vi "Receptor PSK.vi"() -> ()   [LabVIEW 2016]
uses:
  <vilib>/addons/Modulation/Digital/Support/Controls/Pack Bits Parameters.ctl
  <vilib>/addons/Modulation/Analog/support/mod_Set Error Source.vi
  <vilib>/addons/Modulation/Analog/support/Validators/mod_Fractional Resample Validate.vi
  <vilib>/addons/Modulation/Analog/support/Validators/mod_Check Flush State.vi
  <vilib>/addons/Modulation/Analog/support/mod_FractionalResampler.vi
  <vilib>/addons/Modulation/Analog/support/mod_Integer Rate Interpolation.vi
  <vilib>/addons/Modulation/Analog/support/Validators/mod_Validate Complex Waveform.vi
  <vilib>/addons/Modulation/Analog/support/mod_PerformResampling.vi
  <vilib>/addons/Modulation/Analog/support/Validators/mod_WFErrorHandler.vi
  <vilib>/addons/Modulation/Digital/Support/Common/Validators/mod_Generate Filter Coefficients Validate.vi
  <vilib>/addons/Modulation/Digital/General/subVIs/mod_Generate Filter Coefficients.vi
  <instrlib>/niUSRP/niUSRP Fetch Rx Data (CDB Cluster).vi
  <vilib>/addons/Modulation/Digital/General/MT Generate PSK System Parameters(M).vi
  <vilib>/addons/Modulation/Digital/General/MT Generate PSK Synchronization Parameters (bit array).vi
  <vilib>/Utility/error.llb/Error Cluster From Error Code.vi
  <vilib>/addons/Modulation/Analog/support/mod_Resampling Factors.vi
  <vilib>/addons/Modulation/Analog/support/mod_ResamplingFilter.vi
  <vilib>/addons/Modulation/Analog/support/mod_Generate Integer Interpolation Filter.vi
  <instrlib>/niUSRP/niUSRP Fetch Rx Data (CDB WDT).vi
  <vilib>/measure/maspectr.llb/FFT Spectrum (Mag-Phase) for 1 Chan (CDB).vi
  <vilib>/addons/Modulation/niDMT.lvlib
  <vilib>/addons/Modulation/niAMT.lvlib
  <vilib>/measure/NI_MAPro.lvlib
panel:
  in  "Header":u32=10 format="%b"
  out "Symbol rate":dbl
  out "output bit stream":i8[](array[numeric])
  out "Magnitude Spectrum":cluster{"f0":dbl, "df":dbl, "magnitude":dbl[]}(graph)={"f0"=-100000.0, "df"=20.0, "magnitude"=[]}
  out "Acquired Signal":waveform(dbl)[](graph)
  out "Frame Size [samples]":i64=20000
  in  "Acq Duration [sec]":dbl=0.01 format="%#.6p"
  in  "autoscale":bool
  out "Constellation Graph":T1(graph)
  in  "stop":bool
  out "measurements":T2={"frequency offset (Hz)"=-11.93165072236316, "frequency drift (Hz)"=0.08770196207837619, "phase offset (deg)"=52.673364140832604} {"phase offset (deg)" format="%.2f"; "frequency drift (Hz)" format="%.2f"; "frequency offset (Hz)" format="%.2f"}
  in  "filter parameters":T3={"Alpha"=0.5, "Filter Length"=6, "TX Filter"=enum."Root Raised Cos"} {"Alpha" format="%.2f"}
  out "Gain [dB] (actual)":dbl=12.0 format="%#.6p"
  out "Carrier Frequency \n[Hz] (actual)":dbl=915000000.0 format="%#.6p"
  out "IQ Sampling\nRate [S/sec] (actual)":dbl=500000.0 format="%#.6p"
  in  "Active Antenna":string(combo)="RX1"
  in  "Gain [dB]":dbl=12.0 format="%#.6p"
  in  "Carrier\nFrequency [Hz]":dbl=915000000.0 format="%#.6p"
  in  "IQ Sampling\nRate [S/sec]":dbl=500000.0 format="%#.6p"
  out "session handle out":refnum<k15>
  in  "error in (no error)":errorcluster
  in  "device names":refnum<k15>
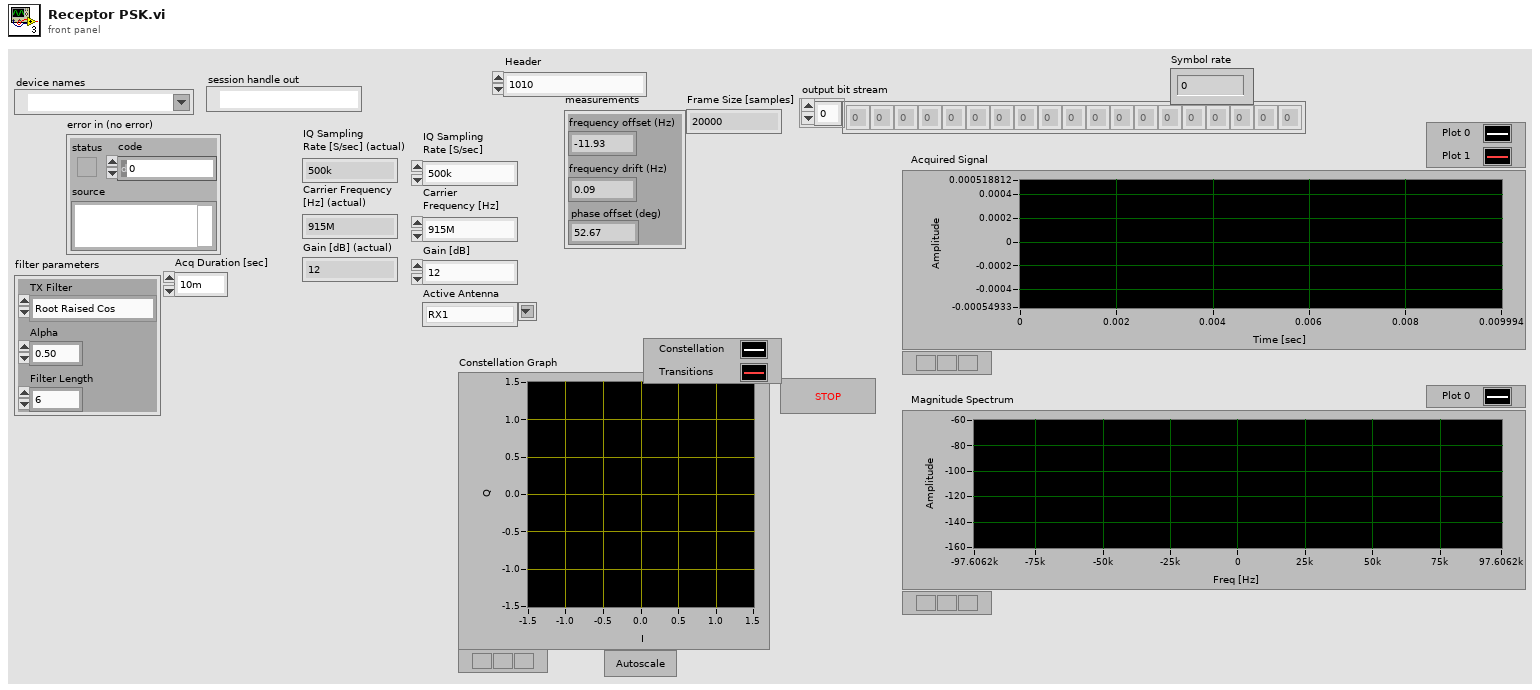
[diagram p1: front panel]
types:
  T1 = cluster{"Decimated Array":dbl[], "Decimated Array":dbl[]}[]
  T2 = cluster{"frequency offset (Hz)":dbl, "frequency drift (Hz)":dbl, "phase offset (deg)":dbl}
  T3 = cluster{"Alpha":dbl, "Filter Length":i32, "TX Filter":enum16{"none", "Raised Cosine", "Root Raised Cos", "Gaussian"}}
  T4 = typedef "niDMT.lvlib/Pack Bits Parameters.ctl" = enum16{"Unsigned", "Signed"}
  T5 = enum16{"FSK", "PSK", "QAM", "MSK", "PAM", "ASK", "CPM"}
  T6 = enum16{"none", "Raised Cosine", "Root Raised Cos", "Gaussian"}
  T7 = cluster{"samples per symbol (16)":i32, "symbol map":cdb[], "differential PSK":enum16{"disable", "enable"}, "PSK type":u16}
  T8 = cluster{"expected sync location (symbols)":i32, "sync sequence":cdb[], "sync location uncertainty (symbols)":i32, "sync indent (symbols)":i32}
  T9 = cluster{"dB On (F)":bool, "unwrap phase (F)":bool, "convert to degree (F)":bool}
  T10 = typedef "niAMT.lvlib/Complex Data Waveform.ctl" = cluster{"t0":dbl, "dt":dbl, "Y":cdb[]}
  T11 = cluster{"constellation":dbl[], "oversampled data":dbl[]}[]
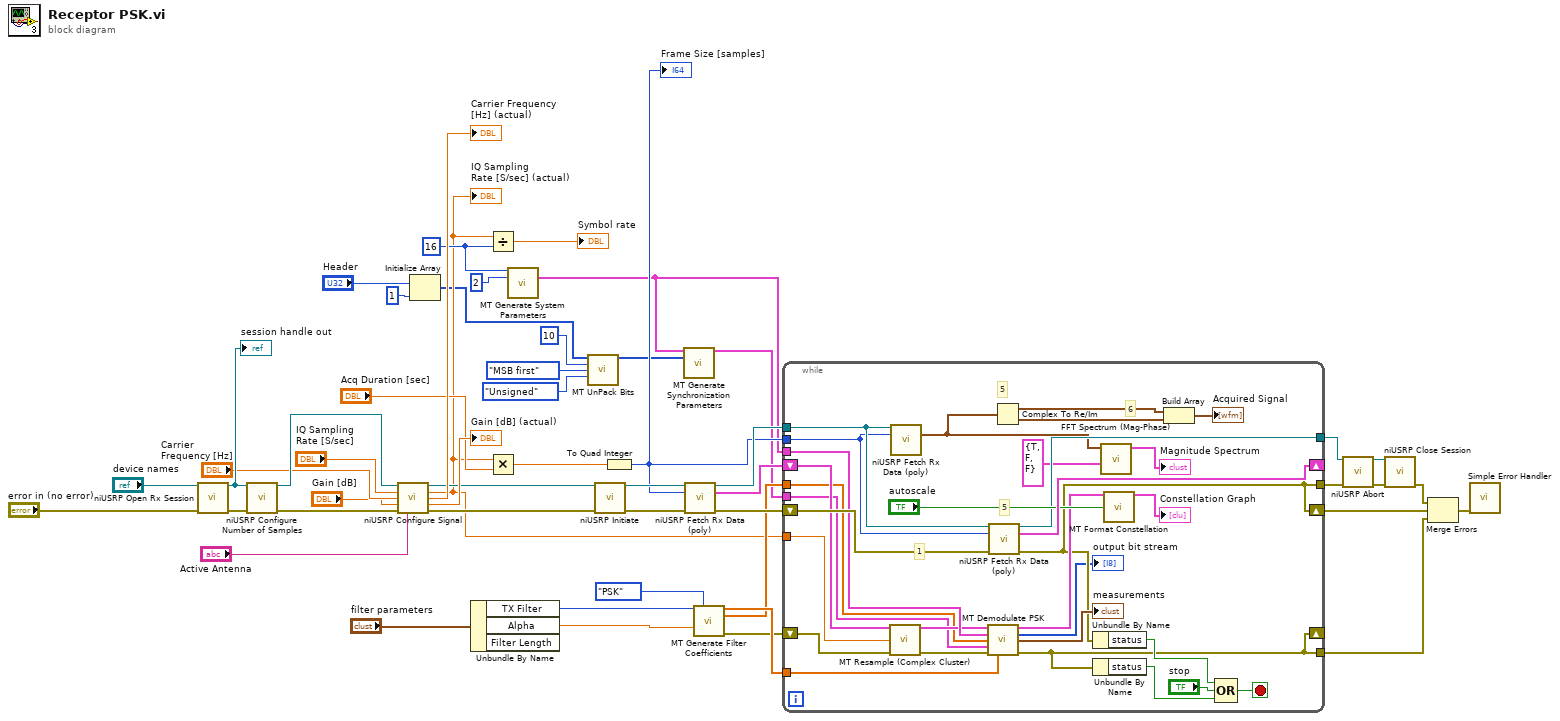
[diagram p0: block diagram]
diagram:
  w11 = 16 ("samples per symbol (16)")
  n1 = call <instrlib>:"niUSRP Open Rx Session.vi"("device names"="device names", "error in (no error)"="error in (no error)") -> ("session handle out"=w48:refnum<k15>, "error out"=w47:errorcluster)  [unwired: 12 in]
  "session handle out" <- w48
  n2 = call <instrlib>:"niUSRP Configure Number of Samples.vi"("session handle"=w48, "error in (no error)"=w47) -> ("session handle out"=w46:refnum<k15>, "error out"=w41:errorcluster)  [unwired: 12 in]
  n3 = call <instrlib>:"niUSRP Configure Signal.vi"("session handle"=w46, "IQ rate"="IQ Sampling\nRate [S/sec]", "carrier frequency"="Carrier\nFrequency [Hz]", "gain"="Gain [dB]", "error in (no error)"=w41, "active antenna"="Active Antenna") -> ("session handle out"=w38:refnum<k15>, "coerced IQ rate"=w10:dbl, "coerced carrier frequency"=→"Carrier Frequency \n[Hz] (actual)":dbl, "coerced gain"=→"Gain [dB] (actual)":dbl, "error out"=w37:errorcluster)  [unwired: 5 in]
  "IQ Sampling\nRate [S/sec] (actual)" <- w10
  n4 = Initialize Array("Header", 1 ("dimension size")) -> (w3:u32[])
  n5 = Unbundle By Name("filter parameters") -> ("TX Filter"=w31:T6, "Alpha"=w32:dbl)  [unwired: 1 out]
  n6 = Divide(x=w10, y=w11) -> (x/y=→"Symbol rate":dbl)
  n7 = Multiply(x=w10, y="Acq Duration [sec]") -> (x*y=w24:dbl)
  n8 = call-poly <vilib>:"MT Generate System Parameters.vi"("samples per symbol (16)"=w11, "M-PSK (4)"=2) -> ("PSK system parameters"=w9:T7)  [unwired: 11 in, 2 out]
  n9 = call <vilib>:"MT UnPack Bits.vi"("input integers"=w3, "bits per integer"=10, "packed bit order"=enum16{"MSB first", "LSB first"}."MSB first", "integer format"=Pack_Bits_Parameters."Unsigned") -> ("output bit stream"=w1:i8[])  [unwired: 10 in, 1 out]
  n10 = call <instrlib>:"niUSRP Initiate.vi"("session handle"=w38, "error in (no error)"=w37) -> ("session handle out"=w36:refnum<k15>, "error out"=w35:errorcluster)  [unwired: 12 in]
  n11 = To Quad Integer(1:w24) -> (0:w23:i64)
  "Frame Size [samples]" <- w23
  n12 = call-poly <vilib>:"MT Generate Synchronization Parameters.vi"("PSK system parameters"=w9, "sync bits"=w1) -> ("PSK synchronization parameters"=w8:T8)  [unwired: 12 in, 1 out]
  n13 = call-poly <instrlib>:"niUSRP Fetch Rx Data (poly).vi"("session handle"=w36, "number of samples"=w23, "error in (no error)"=w35) -> ("session handle out"=w29:refnum<k15>, "data"=w27:cluster{"t0":dbl, "dt":dbl, "Y":cdb[]}, "error out"=w28:errorcluster)  [unwired: 9 in, 1 out]
  n14 = call <vilib>:"MT Generate Filter Coefficients.vi"("pulse shaping filter (none)"=w31, "modulation type"=T5."PSK", "filter parameter"=w32) -> ("pulse shaping filter coefficients"=w26:dbl[], "matched filter coefficients"=w13:dbl[], "error out"=w25:errorcluster)  [unwired: 10 in]
  n15 = while {
    tunnel: w29 -> [w61]
    shift-right: [w65] -> w17
    shift-left: w28 -> [w81]
    shift-right: [w80] -> _
    shift-left: w27 -> [w77]
    tunnel: w26 -> [w79]
    tunnel: w9 -> [w78]
    shift-right: [w63] -> _
    shift-left: w25 -> [w76]
    tunnel: w23 -> [w60]
    tunnel: [w65] -> w16
    tunnel: [w64] -> w15
    tunnel: [w63] -> w14
    tunnel: w13 -> [w62]
    tunnel: w10 -> [w52]
    tunnel: w8 -> [w51]
    stop <- w72 stop-if-true
    # "6"
    # "5"
    # "5"
    # "1"
    n16 = call <vilib>:"MT Resample (Complex Cluster).vi"("input complex waveform"=w77, "desired sample rate (Hz)"=w52, "error in (no error)"=w76) -> ("output complex waveform"=w74:T10, "error out"=w75:errorcluster)  [unwired: 11 in]
    n17 = call-poly <instrlib>:"niUSRP Fetch Rx Data (poly).vi"("session handle"=w61, "number of samples"=w60) -> ("data"=w54:waveform(cdb))  [unwired: 10 in, 3 out]
    n18 = call <vilib>:"MT Demodulate PSK.vi"("input complex waveform"=w74, "PSK system parameters"=w78, "matched filter coefficients"=w62, "synchronization parameters"=w51, "error in (no error)"=w75, "pulse shaping filter coefficients"=w79) -> ("recovered complex waveform"=w67:T10, "output bit stream"=→"output bit stream":i8[], "measurements"=→"measurements":T2, "error out"=w63:errorcluster)  [unwired: 5 in, 1 out]
    n19 = call-poly <instrlib>:"niUSRP Fetch Rx Data (poly).vi"("session handle"=w61, "number of samples"=w60, "error in (no error)"=w81) -> ("session handle out"=w64:refnum<k15>, "data"=w80:cluster{"t0":dbl, "dt":dbl, "Y":cdb[]}, "error out"=w65:errorcluster)  [unwired: 9 in, 1 out]
    n20 = Complex To Re/Im(x + iy=w54) -> (x=w57:waveform(dbl), y=w56:waveform(dbl))
    n21 = Unbundle By Name(w65) -> ("status"=w68:bool)
    n22 = Unbundle By Name(w63) -> ("status"=w69:bool)
    n23 = call-poly <vilib>:"FFT Spectrum (Mag-Phase).vi"("view"=T9 {"dB On (F)"=TRUE, "unwrap phase (F)"=FALSE, "convert to degree (F)"=FALSE}, "time signal"=w54) -> ("magnitude"=→"Magnitude Spectrum":cluster{"f0":dbl, "df":dbl, "magnitude":dbl[]})  [unwired: 5 in, 4 out]
    n24 = call <vilib>:"MT Format Constellation.vi"("waveform"=w67, "autoscale"="autoscale") -> ("constellation graph"=→"Constellation Graph":T11)  [unwired: 12 in, 1 out]
    n25 = Build Array(w57, w56) -> (→"Acquired Signal":waveform(dbl)[])
    n26 = Compound Arithmetic op=OR(w68, "stop", w69) -> (w72:bool)
  }
  n27 = call <instrlib>:"niUSRP Abort.vi"("session handle"=w15, "error in (no error)"=w16) -> ("session handle out"=w20:refnum<k15>, "error out"=w19:errorcluster)  [unwired: 12 in]
  n28 = call <instrlib>:"niUSRP Close Session.vi"("session handle"=w20, "error in (no error)"=w19) -> ("error out"=w18:errorcluster)  [unwired: 13 in]
  n29 = Merge Errors(w18, w17, w14) -> (w21:errorcluster)
  n30 = call <vilib>:"Simple Error Handler.vi"("error in (no error)"=w21) -> ()  [unwired: 4 in, 5 out]
